vi "testScript.vi"() -> ()   [LabVIEW 2017]
panel:
  out "vector restricted 4":i32[](array[numeric])
  out "x > 0?":bool
  out "vector restricted 3":i32[](array[numeric])
  out "vector restricted 2":i32[](array[numeric])
  out "Platforms \nto raise":i32[](array[numeric])
  out "Array 2":i32[](array[numeric])
  out "output":u32[](array[numeric])
  out "vector restricted":i32[](array[numeric])
  out "distance of \nchoices":i32[](array[numeric])
  out "distance":i32
  out "platform choices":i32[](array[numeric])
  in  "previousChoices":i32[][](array[numeric])
  in  "Goal \nplatform":i32
  in  "Start platform":i32
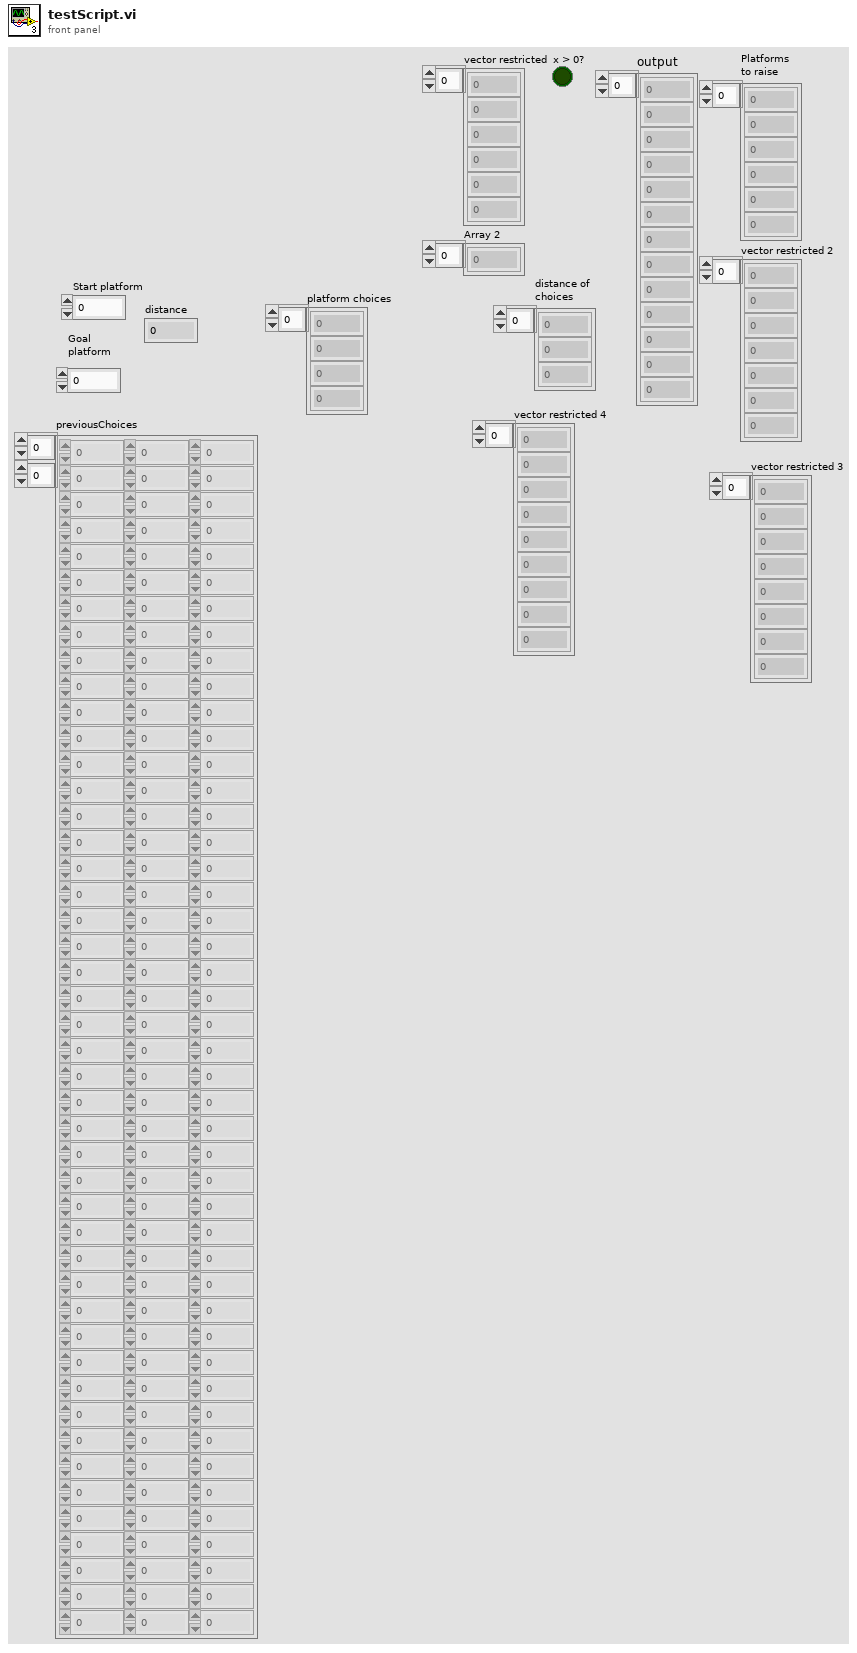
[diagram p1: front panel]
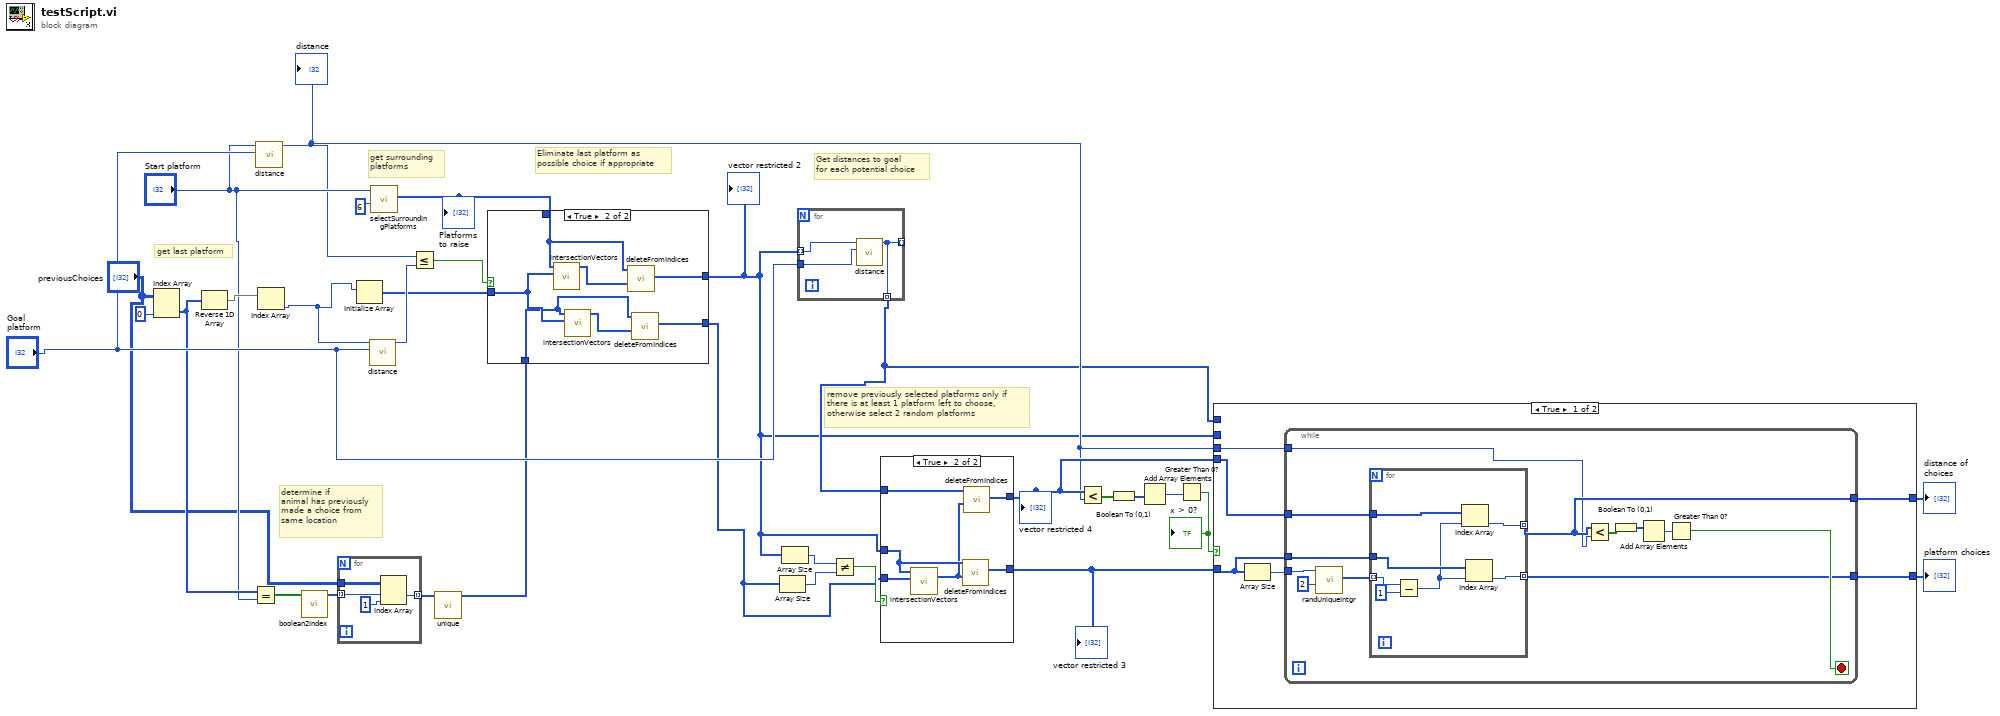
[diagram p0: block diagram]
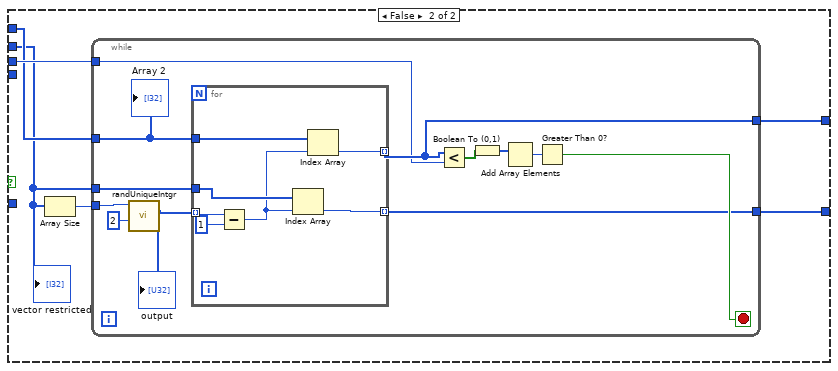
[diagram p2: hidden frame]
diagram:
  # "remove previously selected platforms only if \nthere is at least 1 platform left to choose,\notherwise select 2 random platforms"
  # "determine if \nanimal has previously \nmade a choice from \nsame location"
  # "Get distances to goal\nfor each potential choice"
  # "Eliminate last platform as \npossible choice if appropriate"
  # "get last platform"
  # "get surrounding\nplatforms"
  n1 = Index Array(array="previousChoices", index (col)=0 ("disabled index (col)")) -> (element=w19:i32[])  [unwired: 1 in]
  n2 = Reverse 1D Array(array=w19) -> (reversed array=w29:i32[])
  n3 = Equal?(x=w19, y="Start platform") -> (x = y?=w23:bool[])
  n4 = call "distance.vi"("Goal \nplatform"="Goal \nplatform", "Start \nplatform"="Start platform") -> ("distance"=w5:i32)  [unwired: 9 in]
  "distance" <- w5
  n5 = Index Array(array=w29) -> (element=w26:i32)  [unwired: 1 in]
  n6 = call "boolean2Index.vi"("boolean"=w23) -> ("index"=w22:i32[])  [unwired: 10 in]
  n7 = for {
    tunnel: w22 -> [w34] mode=indexing
    tunnel: "previousChoices" -> [w35]
    tunnel: [w32] -> w16 mode=indexing
    n8 = Index Array(array=w35, index (row)=w34, index (col)=1) -> (element=w32:i32)
  }
  n9 = Initialize Array(w26) -> (w25:i32[])  [unwired: 1 in]
  n10 = call "distance.vi"("Goal \nplatform"="Goal \nplatform", "Start \nplatform"=w26) -> ("distance"=w28:i32)  [unwired: 9 in]
  n11 = call "selectSurroundingPlatforms.vi"("Number of surrounding\nplatforms to raise"=6 ("Number of surrounding\nplatforms to raise"), "Start platform"="Start platform") -> ("Platforms \nto raise"=w15:i32[])  [unwired: 9 in]
  "Platforms \nto raise" <- w15
  n12 = Less Or Equal?(x=w5, y=w28) -> (x <= y?=w27:bool)
  n13 = call "unique.vi"("Array"=w16) -> ("Array 2"=w14:i32[])  [unwired: 10 in]
  n14 = case shown="True" w27 {
    tunnel: w15 -> [w37 w43]
    tunnel: w25 -> [_ w41]
    tunnel: [w37 w42] -> w3
    tunnel: w14 -> [w36 w39]
    tunnel: [w36 w38] -> w11
    frame False {
    }
    frame True {
      n15 = call "intersectionVectors.vi"("vector2"=w41, "vector1"=w43) -> ("vector1 indices"=w44:i32[])  [unwired: 8 in, 1 out]
      n16 = call "intersectionVectors.vi"("vector2"=w41, "vector1"=w39) -> ("vector1 indices"=w40:i32[])  [unwired: 8 in, 1 out]
      n17 = call "deleteFromIndices.vi"("indices to delete"=w44, "vector"=w43) -> ("vector restricted"=w42:i32[])  [unwired: 9 in]
      n18 = call "deleteFromIndices.vi"("indices to delete"=w40, "vector"=w39) -> ("vector restricted"=w38:i32[])  [unwired: 9 in]
    }
  }
  "vector restricted 2" <- w3
  n19 = Array Size(array=w11) -> (size(s)=w20:i32)
  n20 = Array Size(array=w3) -> (size(s)=w21:i32)
  n21 = for {
    tunnel: w3 -> [w47] mode=indexing
    tunnel: "Goal \nplatform" -> [w46]
    tunnel: [w45] -> _ mode=indexing
    tunnel: [w45] -> w4 mode=indexing
    n22 = call "distance.vi"("Goal \nplatform"=w46, "Start \nplatform"=w47) -> ("distance"=w45:i32)  [unwired: 9 in]
  }
  n23 = Not Equal?(x=w21, y=w20) -> (x != y?=w12:bool)
  n24 = case shown="True" w12 {
    tunnel: [w49 w55] -> w13
    tunnel: w3 -> [w49 w54]
    tunnel: w11 -> [_ w53]
    tunnel: w4 -> [w48 w52]
    tunnel: [w48 w50] -> w6
    frame False {
    }
    frame True {
      n25 = call "intersectionVectors.vi"("vector2"=w53, "vector1"=w54) -> ("vector1 indices"=w51:i32[])  [unwired: 8 in, 1 out]
      n26 = call "deleteFromIndices.vi"("indices to delete"=w51, "vector"=w54) -> ("vector restricted"=w55:i32[])  [unwired: 9 in]
      n27 = call "deleteFromIndices.vi"("indices to delete"=w51, "vector"=w52) -> ("vector restricted"=w50:i32[])  [unwired: 9 in]
    }
  }
  "vector restricted 3" <- w13
  "vector restricted 4" <- w6
  n28 = Less?(x=w6, y=w5) -> (x < y?=w10:bool[])
  n29 = Boolean To (0,1)(Boolean=w10) -> (0, 1=w8:i16[])
  n30 = Add Array Elements(numeric array=w8) -> (sum=w9:i16)
  n31 = Greater Than 0?(x=w9) -> (x > 0?=w7:bool)
  "x > 0?" <- w7
  n32 = case shown="True" w7 {
    tunnel: w13 -> [w60 _]
    tunnel: w6 -> [w59 _]
    tunnel: w5 -> [w58 w85]
    tunnel: [w57 w84] -> w2
    tunnel: w4 -> [_ w83]
    tunnel: w3 -> [_ w82]
    tunnel: [w56 w81] -> w1
    frame True {
      n33 = Array Size(array=w60) -> (size(s)=w61:i32)
      n34 = while {
        tunnel: w61 -> [w73]
        tunnel: w60 -> [w70]
        tunnel: w59 -> [w69]
        tunnel: w58 -> [w62]
        tunnel: [w64] -> w57
        tunnel: [w63] -> w56
        stop <- w65 stop-if-true
        n35 = call "randUniqueIntgr.vi"("max rand number"=w73, "Number of Outputs"=2) -> ("output"=w71:u32[])  [unwired: 8 in]
        n36 = for {
          tunnel: w71 -> [w76] mode=indexing
          tunnel: w70 -> [w80]
          tunnel: w69 -> [w79]
          tunnel: [w78] -> w63 mode=indexing
          tunnel: [w77] -> w64 mode=indexing
          n37 = Subtract(x=w76, y=u32 1) -> (x-y=w75:u32)
          n38 = Index Array(array=w79, index=w75) -> (element=w78:i32)
          n39 = Index Array(array=w80, index=w75) -> (element=w77:i32)
        }
        n40 = Less?(x=w63, y=w62) -> (x < y?=w66:bool[])
        n41 = Boolean To (0,1)(Boolean=w66) -> (0, 1=w68:i16[])
        n42 = Add Array Elements(numeric array=w68) -> (sum=w67:i16)
        n43 = Greater Than 0?(x=w67) -> (x > 0?=w65:bool)
      }
    }
    frame False {
      n44 = Array Size(array=w82) -> (size(s)=w86:i32)
      n45 = while {
        tunnel: w86 -> [w98]
        tunnel: w82 -> [w95]
        tunnel: w83 -> [w94]
        tunnel: w85 -> [w87]
        tunnel: [w89] -> w84
        tunnel: [w88] -> w81
        stop <- w90 stop-if-true
        n46 = call "randUniqueIntgr.vi"("max rand number"=w98, "Number of Outputs"=2) -> ("output"=w96:u32[])  [unwired: 8 in]
        "output" <- w96
        n47 = for {
          tunnel: w96 -> [w101] mode=indexing
          tunnel: w95 -> [w105]
          tunnel: w94 -> [w104]
          tunnel: [w103] -> w88 mode=indexing
          tunnel: [w102] -> w89 mode=indexing
          n48 = Subtract(x=w101, y=u32 1) -> (x-y=w100:u32)
          n49 = Index Array(array=w105, index=w100) -> (element=w102:i32)
          n50 = Index Array(array=w104, index=w100) -> (element=w103:i32)
        }
        n51 = Less?(x=w88, y=w87) -> (x < y?=w91:bool[])
        n52 = Boolean To (0,1)(Boolean=w91) -> (0, 1=w93:i16[])
        n53 = Add Array Elements(numeric array=w93) -> (sum=w92:i16)
        n54 = Greater Than 0?(x=w92) -> (x > 0?=w90:bool)
        "Array 2" <- w94
      }
      "vector restricted" <- w82
    }
  }
  "platform choices" <- w2
  "distance of \nchoices" <- w1
